vi "Lift Back Arms (Darius + Allen).vi"(8 "Constant motor speed":dbl, 9 "reset(default false)":bool, 10 "Encoder distance":dbl, 11 "Desired distance":dbl) -> (0 "move done":bool)   [LabVIEW 2014]
panel:
  out "Enum":T1(ring)
  # "starts again from check\nreseting the program"
  # "In inches,from bottom\n(Or any other unit, so long as both are the same"
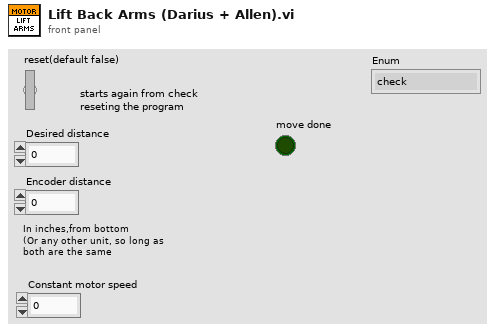
[diagram p1: front panel]
types:
  T1 = enum16{"check", "move up", "move down", "stop move", ""}
  T2 = typedef "WPI_MotorControlDeviceRef.ctl" = cluster{"DeviceStatus":errorcluster, "Type":T3, "PWM":cluster{"Controller":T4, "PWM Channel":T5, "DeadBand":T6}, "CAN":cluster{"Device Number":u8, "Control Mode":T7, "Semaphore":T8, "Max Vout":dbl, "TalonSRX Control Mode":T9}, "Invert":bool, "TransformRef":T10, "InvTransformRef":T10}
  T3 = typedef "WPI_MotorControlType.ctl" = enum16{"PWM", "CAN", "CANTalonSRX"}
  T4 = typedef "FPGA_TypedefDigitalModule.ctl" = enum16{"Controller 1"}
  T5 = typedef "FPGA_DIOPWMChannel.ctl" = enum8{"PWM 0", "PWM 1", "PWM 2", "PWM 3", "PWM 4", "PWM 5", "PWM 6", "PWM 7", "PWM 8", "PWM 9", "PWM MXP 0", "PWM MXP 1", "PWM MXP 2", "PWM MXP 3", "PWM MXP 4", "PWM MXP 5", "PWM MXP 6", "PWM MXP 7", "PWM MXP 8", "PWM MXP 9", "Invalid"}
  T6 = typedef "WPI_PWMDeadband.ctl" = cluster{"Name":string, "maxPositivePwm":i32, "minPositivePwm":i32, "centerPwm":i32, "maxNegativePwm":i32, "minNegativePwm":i32, "angularRange":u16}
  T7 = typedef "WPI_CANJaguar_ControlMode.ctl" = enum8{"Percent VBus", "Current", "Speed", "Position", "Voltage"}
  T8 = typedef "Semaphore RefNum" = refnum<k1>
  T9 = typedef "WPI_CANTalonSRX_APIControlMode.ctl" = enum8{"Percent VBus", "Speed", "Position", "Slave", "Unchanged / Invalid"}
  T10 = typedef "WPI_PWMTransform_ConPane.ctl" = refnum<vi>
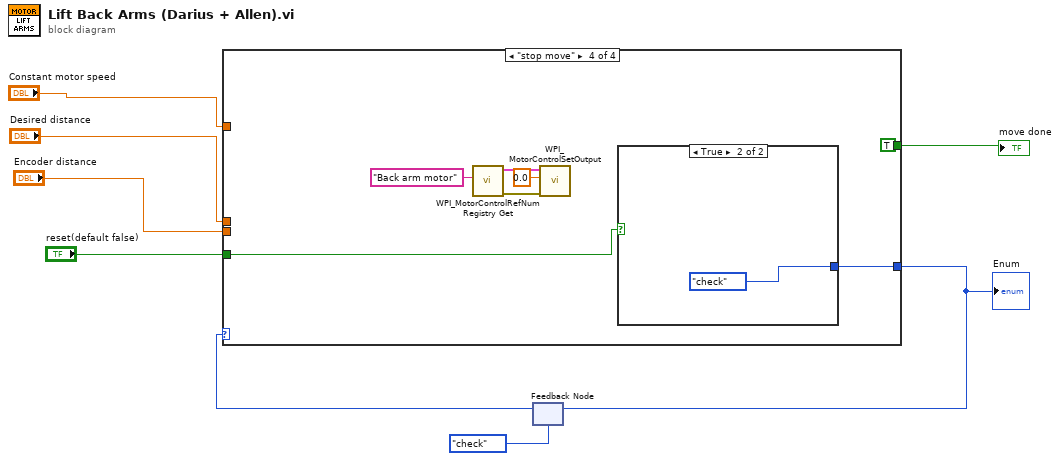
[diagram p0: block diagram]
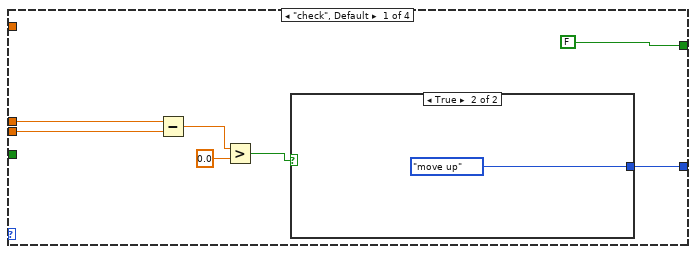
[diagram p2: hidden frame]
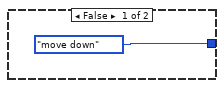
[diagram p3: hidden frame]
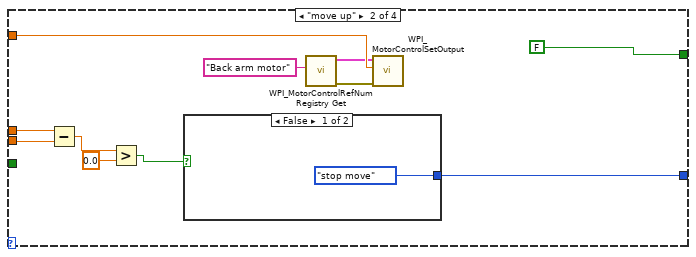
[diagram p4: hidden frame]
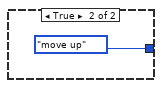
[diagram p5: hidden frame]
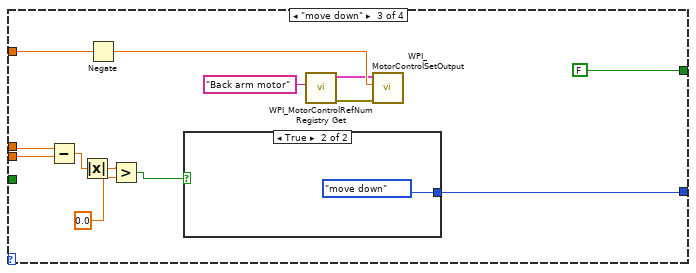
[diagram p6: hidden frame]
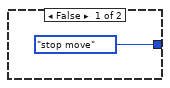
[diagram p7: hidden frame]
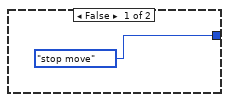
[diagram p8: hidden frame]
diagram:
  n1 = feedback #1(T1."check") -> (w7:T1)
  n2 = case shown="\"stop move\"" w7 {
    tunnel: "Encoder distance" -> [w13 w26 w36 _]
    tunnel: "Desired distance" -> [w12 w27 w37 _]
    tunnel: [w10 w22 w40 w51] -> w6
    tunnel: "Constant motor speed" -> [_ w28 w39 _]
    tunnel: [FALSE FALSE FALSE TRUE] -> w5
    tunnel: "reset(default false)" -> [_ _ _ w46]
    frame "check", Default {
      n3 = Subtract(x=w12, y=w13) -> (x-y=w14:dbl)
      n4 = Greater?(x=w14, y=0.0) -> (0:w11:bool)
      n5 = case shown="True" w11 {
        tunnel: [T1."move down" T1."move up"] -> w10
        frame False {
        }
        frame True {
        }
      }
    }
    frame "move up" {
      n6 = Subtract(x=w27, y=w26) -> (x-y=w25:dbl)
      n7 = Greater?(x=w25, y=0.0) -> (0:w23:bool)
      n8 = case shown="False" w23 {
        tunnel: [T1."stop move" T1."move up"] -> w22
        frame False {
        }
        frame True {
        }
      }
      n9 = call <vilib>:"WPI_MotorControlRefNum Registry Get.vi"("refnum name"="Back arm motor") -> ("error out"=w20:errorcluster, "MotorControlDevRef"=w18:T2)  [unwired: 9 in]
      n10 = call <vilib>:"WPI_MotorControlSetOutput.vi"("error in (no error)"=w20, "Output"=w28, "MotorControlDevRef"=w18) -> ()  [unwired: 6 in, 3 out]
    }
    frame "move down" {
      n11 = Subtract(x=w37, y=w36) -> (x-y=w34:dbl)
      n12 = Absolute Value(x=w34) -> (abs(x)=w35:dbl)
      n13 = Negate(x=w39) -> (-x=w38:dbl)
      n14 = Greater?(x=w35, y=0.0) -> (0:w41:bool)
      n15 = case shown="True" w41 {
        tunnel: [T1."stop move" T1."move down"] -> w40
        frame False {
        }
        frame True {
        }
      }
      n16 = call <vilib>:"WPI_MotorControlRefNum Registry Get.vi"("refnum name"="Back arm motor") -> ("error out"=w33:errorcluster, "MotorControlDevRef"=w31:T2)  [unwired: 9 in]
      n17 = call <vilib>:"WPI_MotorControlSetOutput.vi"("error in (no error)"=w33, "Output"=w38, "MotorControlDevRef"=w31) -> ()  [unwired: 6 in, 3 out]
    }
    frame "stop move" {
      n18 = call <vilib>:"WPI_MotorControlRefNum Registry Get.vi"("refnum name"="Back arm motor") -> ("error out"=w50:errorcluster, "MotorControlDevRef"=w48:T2)  [unwired: 9 in]
      n19 = call <vilib>:"WPI_MotorControlSetOutput.vi"("error in (no error)"=w50, "Output"=0.0, "MotorControlDevRef"=w48) -> ()  [unwired: 6 in, 3 out]
      n20 = case shown="True" w46 {
        tunnel: [T1."stop move" T1."check"] -> w51
        frame False {
        }
        frame True {
        }
      }
    }
  }
  "move done" <- w5
  "Enum" <- w6
  n21 = feedback-in #1(w6) -> ()
